vi "Actor Launched.vi"(5 "Actor's Caller":refnum<class "Message Enqueuer.lvclass">, 6 "Actor Core Name":string, 7 "Actor's Queue":refnum<class "Message Enqueuer.lvclass">, 8 "error in (no error)":errorcluster, 9 "Actor ID":string, 10 "Class Name":string, 11 "Actor Monitor in":refnum<class "Actor Monitor.lvclass">) -> (0 "error out":errorcluster, 3 "Actor Monitor out":refnum<class "Actor Monitor.lvclass">)   [LabVIEW 2018, in "Monitored Actor.lvlib" / "Actor Monitor.lvclass"]
doc: "Adds the new Actor to the proper data structures so we can look it up later.\n\nQueue Lookup By Core Name is used to map a core name to a Queue Object. I use this to send messages to the actor as needed.\n\nNested Actor Lookup is used to determine what actors launch other actors. I use the Actor's Caller Queue to lookup if I have seen it's parent (in terms of nested actors, not inheritance) was a monitored actor. If it is, I add it to the tree under the parent actor.\n\nCopyright: MGI\nAuthored by: Derek Trepanier"
uses:
  Actor Monitor.lvclass
  <vilib>/ActorFramework/Message Enqueuer/Message Enqueuer.lvclass
  UI Info.ctl
  Actor Monitor.lvclass/Actor Monitor.ctl
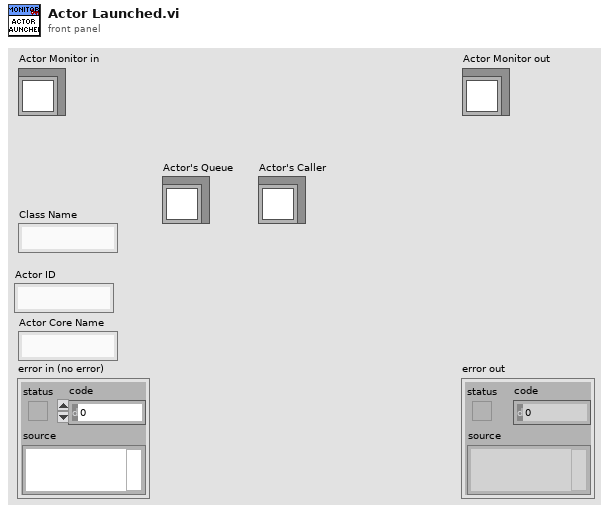
[diagram p1: front panel]
types:
  T1 = typedef "Monitored Actor.lvlib/Actor Monitor.lvclass/UI Info.ctl" = cluster{"Class Name":string, "Actor Core Name":string, "Ping Response Str":string}
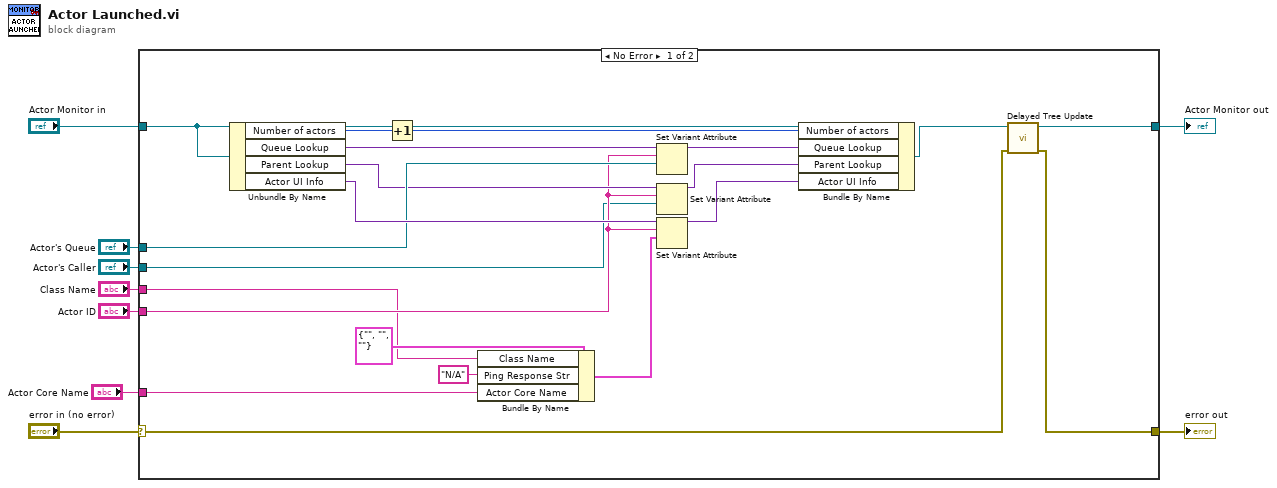
[diagram p0: block diagram]
diagram:
  n1 = case shown="No Error" "error in (no error)" {
    selector: "error in (no error)" -> [w14 w32]
    tunnel: [w13 w32] -> w8
    tunnel: [w15 w31] -> w6
    tunnel: "Actor Monitor in" -> [w30 w31]
    tunnel: "Actor's Caller" -> [w21 _]
    tunnel: "Class Name" -> [w19 _]
    tunnel: "Actor ID" -> [w22 _]
    tunnel: "Actor's Queue" -> [w25 _]
    tunnel: "Actor Core Name" -> [w10 _]
    frame No Error {
      n2 = Unbundle By Name(w30) -> ("Number of actors"=w12:u32, "Queue Lookup"=w27:variant, "Parent Lookup"=w24:variant, "Actor UI Info"=w28:variant)
      n3 = Increment(x=w12) -> (x+1=w11:u32)
      n4 = Bundle By Name(cluster=T1 {"Class Name"="", "Actor Core Name"="", "Ping Response Str"=""} ("UI Info"), "Class Name"=w19, "Ping Response Str"="N/A", "Actor Core Name"=w10) -> (w18:T1)
      n5 = Set Variant Attribute(Variant=w27, name=w22, value=w25) -> (Variant out=w26:variant)  [unwired: 1 in, 2 out]
      n6 = Set Variant Attribute(Variant=w24, name=w22, value=w21) -> (Variant out=w23:variant)  [unwired: 1 in, 2 out]
      n7 = Set Variant Attribute(Variant=w28, name=w22, value=w18) -> (Variant out=w29:variant)  [unwired: 1 in, 2 out]
      n8 = Bundle By Name(cluster=w30, "Number of actors"=w11, "Queue Lookup"=w26, "Parent Lookup"=w23, "Actor UI Info"=w29) -> (w16:refnum<class "Actor Monitor.lvclass">)
      n9 = call "Delayed Tree Update.vi"("error in (no error)"=w14, "Actor Monitor in"=w16) -> ("error out"=w13:errorcluster, "Actor Monitor out"=w15:refnum<class "Actor Monitor.lvclass">)  [unwired: 8 in]
    }
    frame Error {
    }
  }
  "error out" <- w8
  "Actor Monitor out" <- w6
